vi "溶解氧电极校准.vi"() -> ()   [LabVIEW 2016, in "斯坦道多参数.lvlib"]
uses:
  <vilib>/Utility/miscctls.llb/LVPointTypeDef.ctl
  <vilib>/Analysis/NI_AALBase.lvlib
  <vilib>/ptbypt/NI_PtbyPt.lvlib
panel:
  out "标液2":string="饱和标准液"
  out "标液1":string="零点标准液"
  in  "刷新按钮":bool
  out "第二点信号值":dbl
  out "第一点信号值":dbl
  out "通讯状态":string
  out "第二点校准值":dbl
  out "第一点校准值":dbl
  out "最小值":sgl format="%#.2f"
  out "最大值":sgl format="%#.2f"
  in  "校准模式":enum16{"两点校准", "单点校准"}(ring)=enum."单点校准"
  in  "校准停止":bool
  in  "校准启动":bool
  out "波形图表":dbl(graph) caption="历史曲线"
  out "变异系数":dbl format="%#.6f"
  out "standard deviation":dbl caption="标准差" format="%#.2f"
  out "mean":dbl caption="均值" format="%#.2f"
  out "测量读值":dbl caption="测量值" format="%#.2f"
  out "偏移值补偿":dbl caption="溶解氧偏移修正值" format="%#.2f"
  out "饱和度值":dbl format="%#.2f"
  out "提示":string
  out "气压补偿值":dbl format="%#.2f"
  out "盐度补偿值":dbl format="%#.2f"
  out "电极斜率":dbl format="%#.6f"
  out "电极零点":dbl format="%#.6f"
  # "溶解氧电极设定"
  # "%"
  # "%"
  # "ppt"
  # "hPa"
  # "请选择校准模式:"
  # "mg/L"
  # "%"
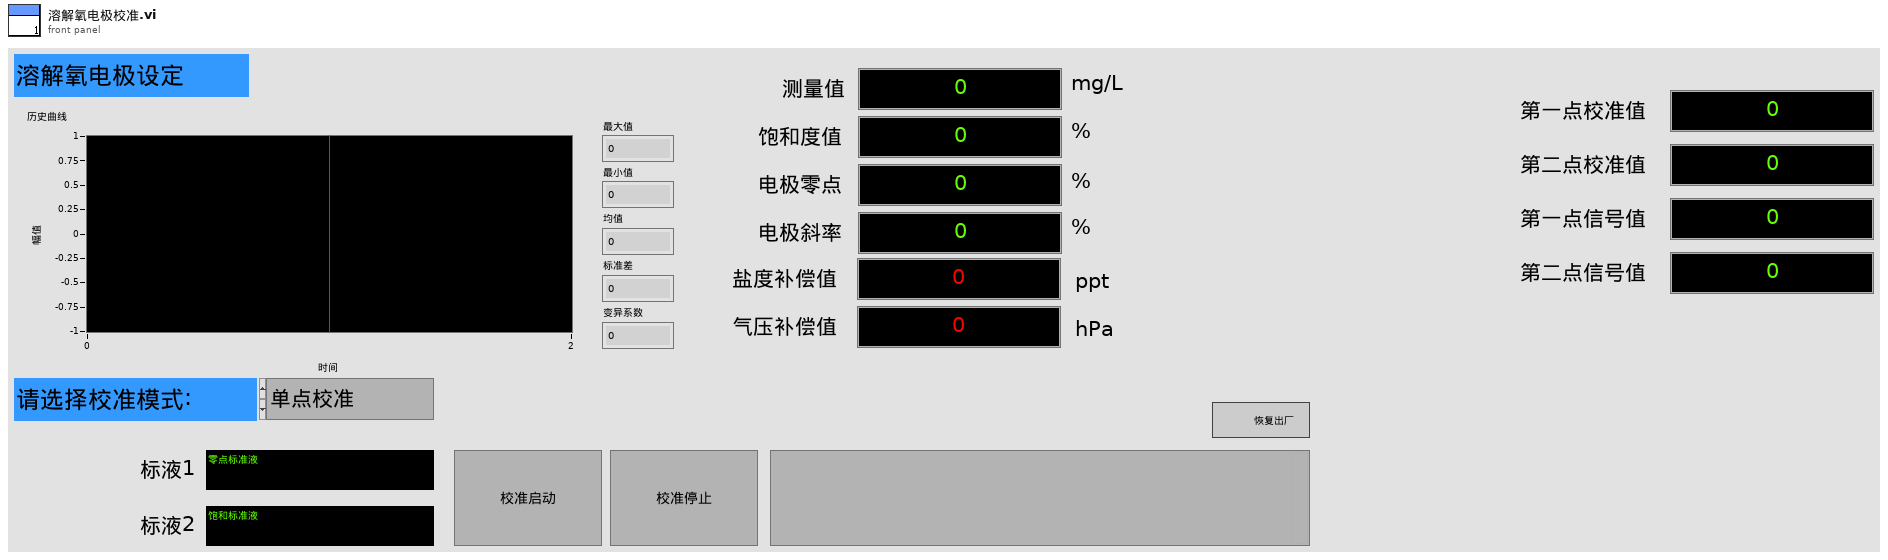
[diagram p1: front panel]
types:
  T1 = typedef "LVPointTypeDef.ctl" = cluster{"Horizontal":i16, "Vertical":i16}
  T2 = cluster{"电极状态标志":u16, "电极型号标志":u16, "溶解氧测量值":sgl, "温度测量值":sgl, "溶解氧饱和度值":sgl, "盐度补偿值":sgl, "大气压补偿值":sgl, "溶解氧偏移修正值":sgl, "温度偏移修正值":sgl, "手动温度补偿值":sgl, "溶解氧电极零点":sgl, "溶解氧电极斜率":sgl, "第1点标准值记录":sgl, "第1点信号值记录":sgl, "第1点温度值记录":sgl, "第2点标准值记录":sgl, "第2点信号值记录":sgl, "第2点温度值记录":sgl, "命令滤波设定":u16, "温度模式":enum16{"ATC", "MTC"}, "生产批次":u16, "电极序号":u16, "串口地址":u16, "串口波特率":enum16{"9600", "19200", "115200"}, "串口校验位":enum16{"NONE", "ODD", "EVEN"}, "串口停止位":enum16{"1bit", "2bit"}, "第一点标准值":sgl, "第二点标准值":sgl}
  T3 = enum8{"Enabled", "Disabled", "Disabled and Grayed Out"}
  T4 = cluster{"ph":bool, "DO":bool, "Cond":bool, "Turb":bool, "叶绿素a":bool, "藻密度":bool, "ORP":bool}
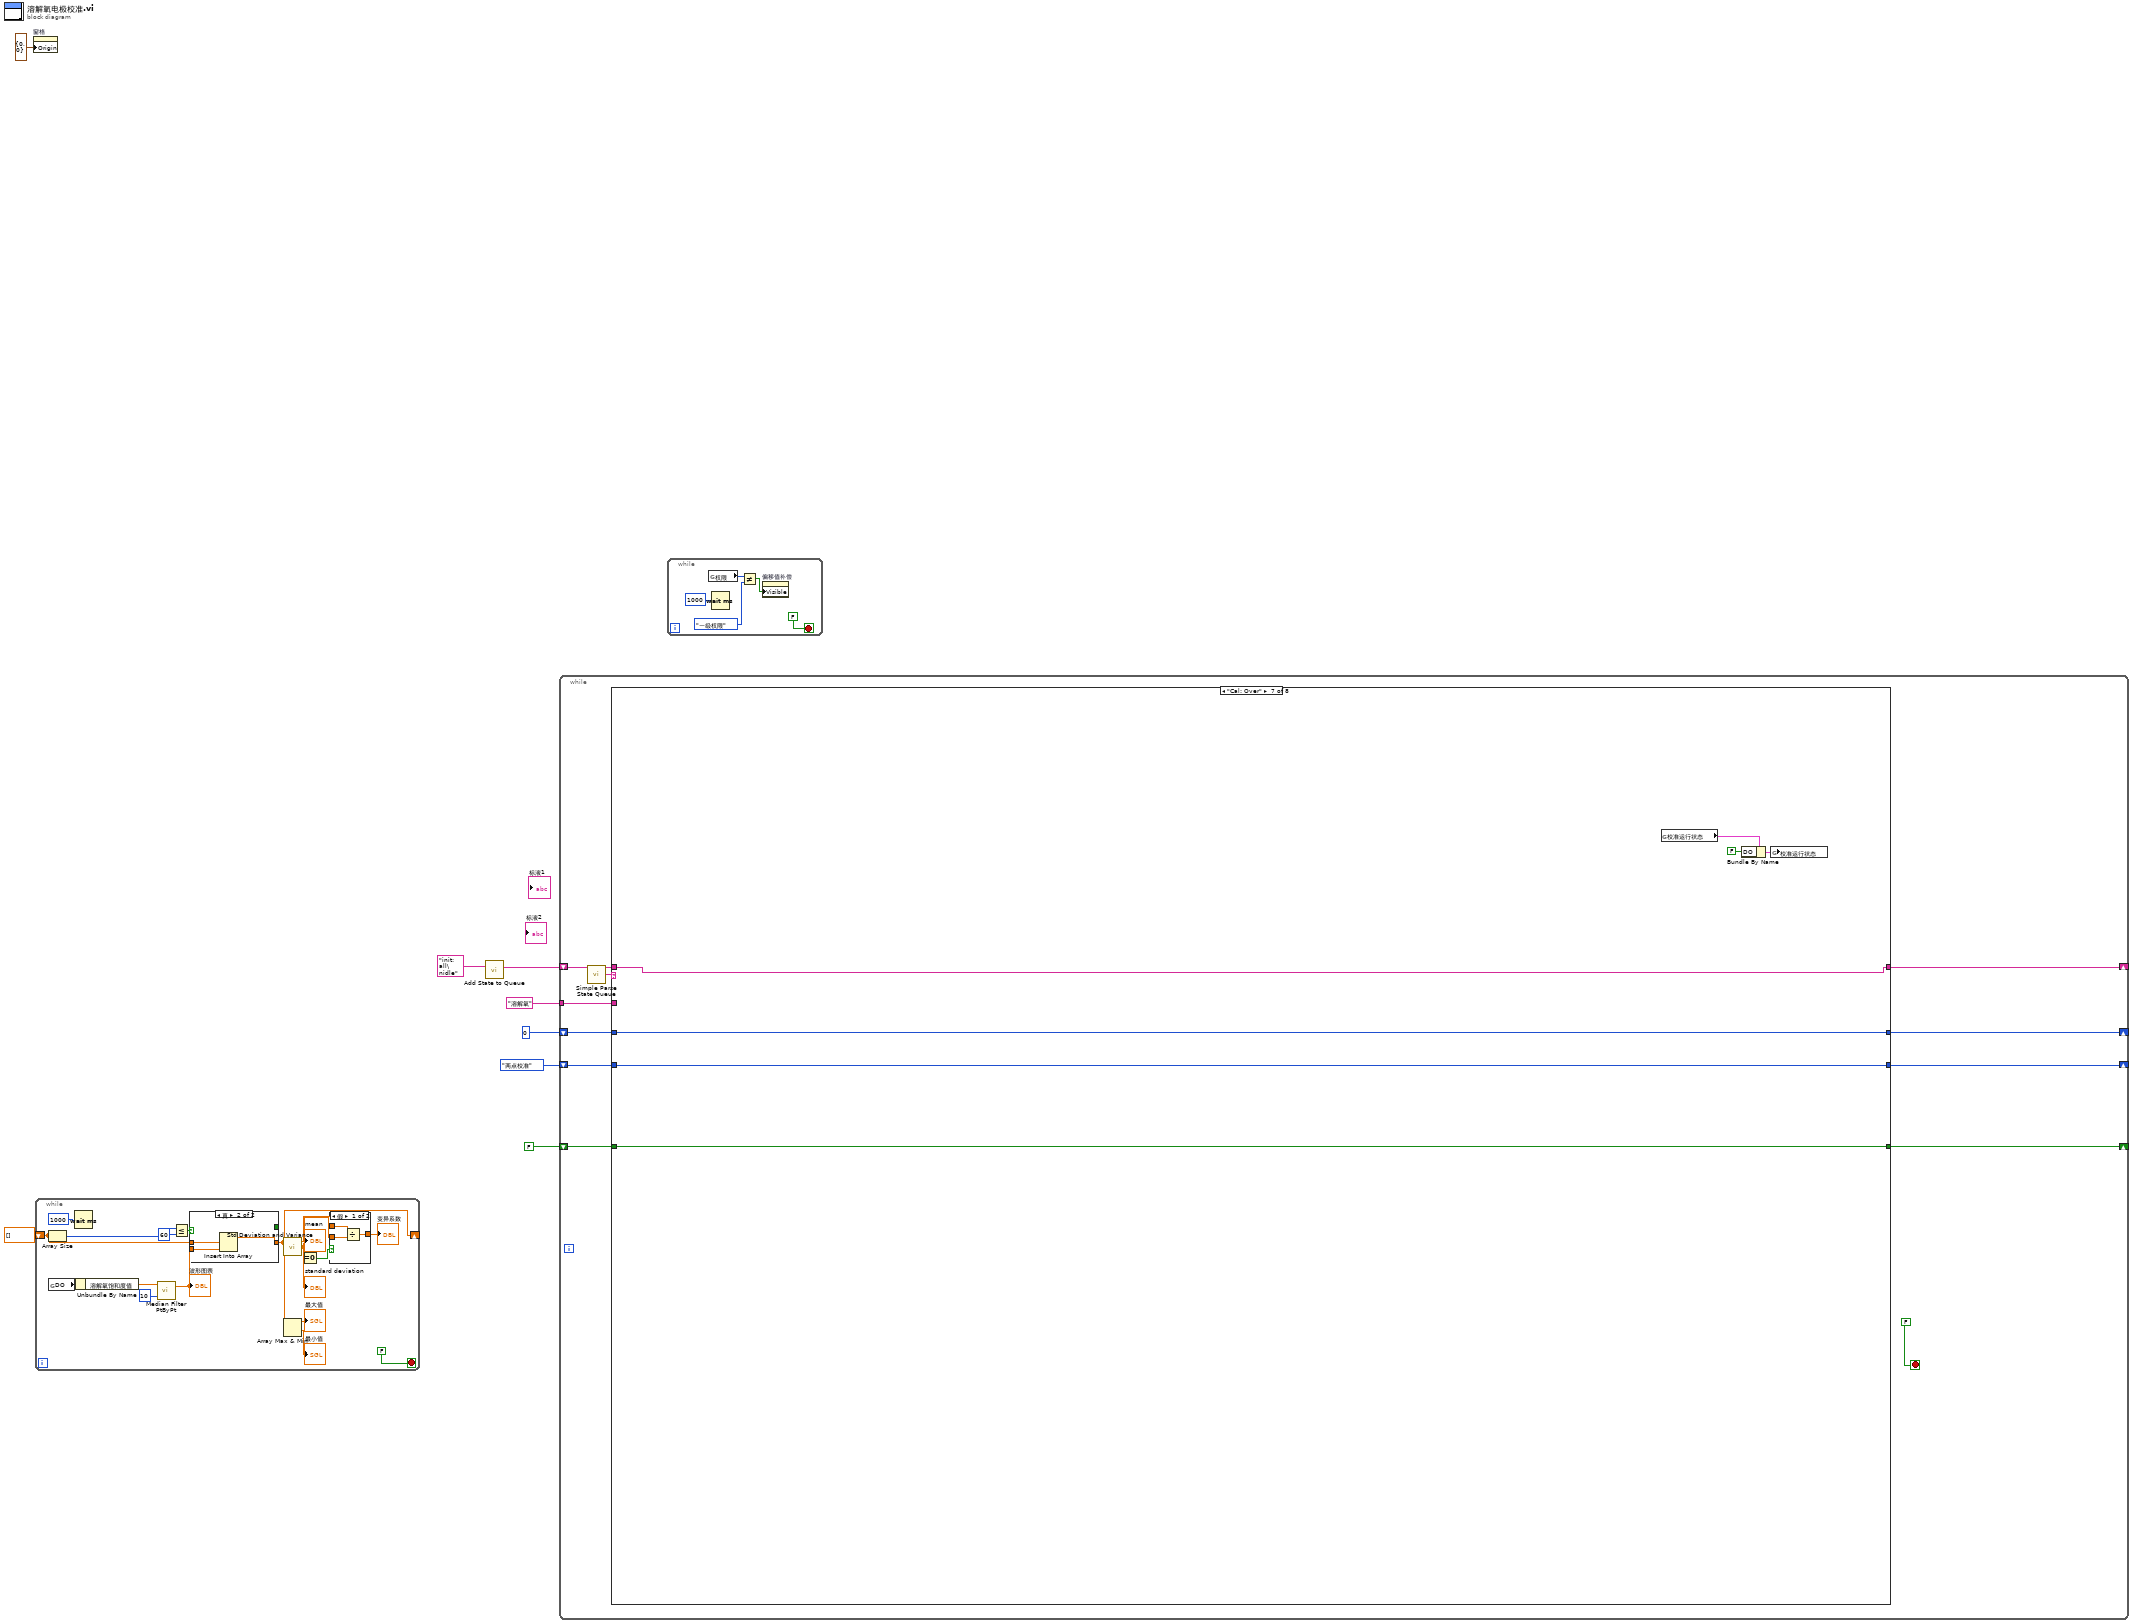
[diagram p0: block diagram]
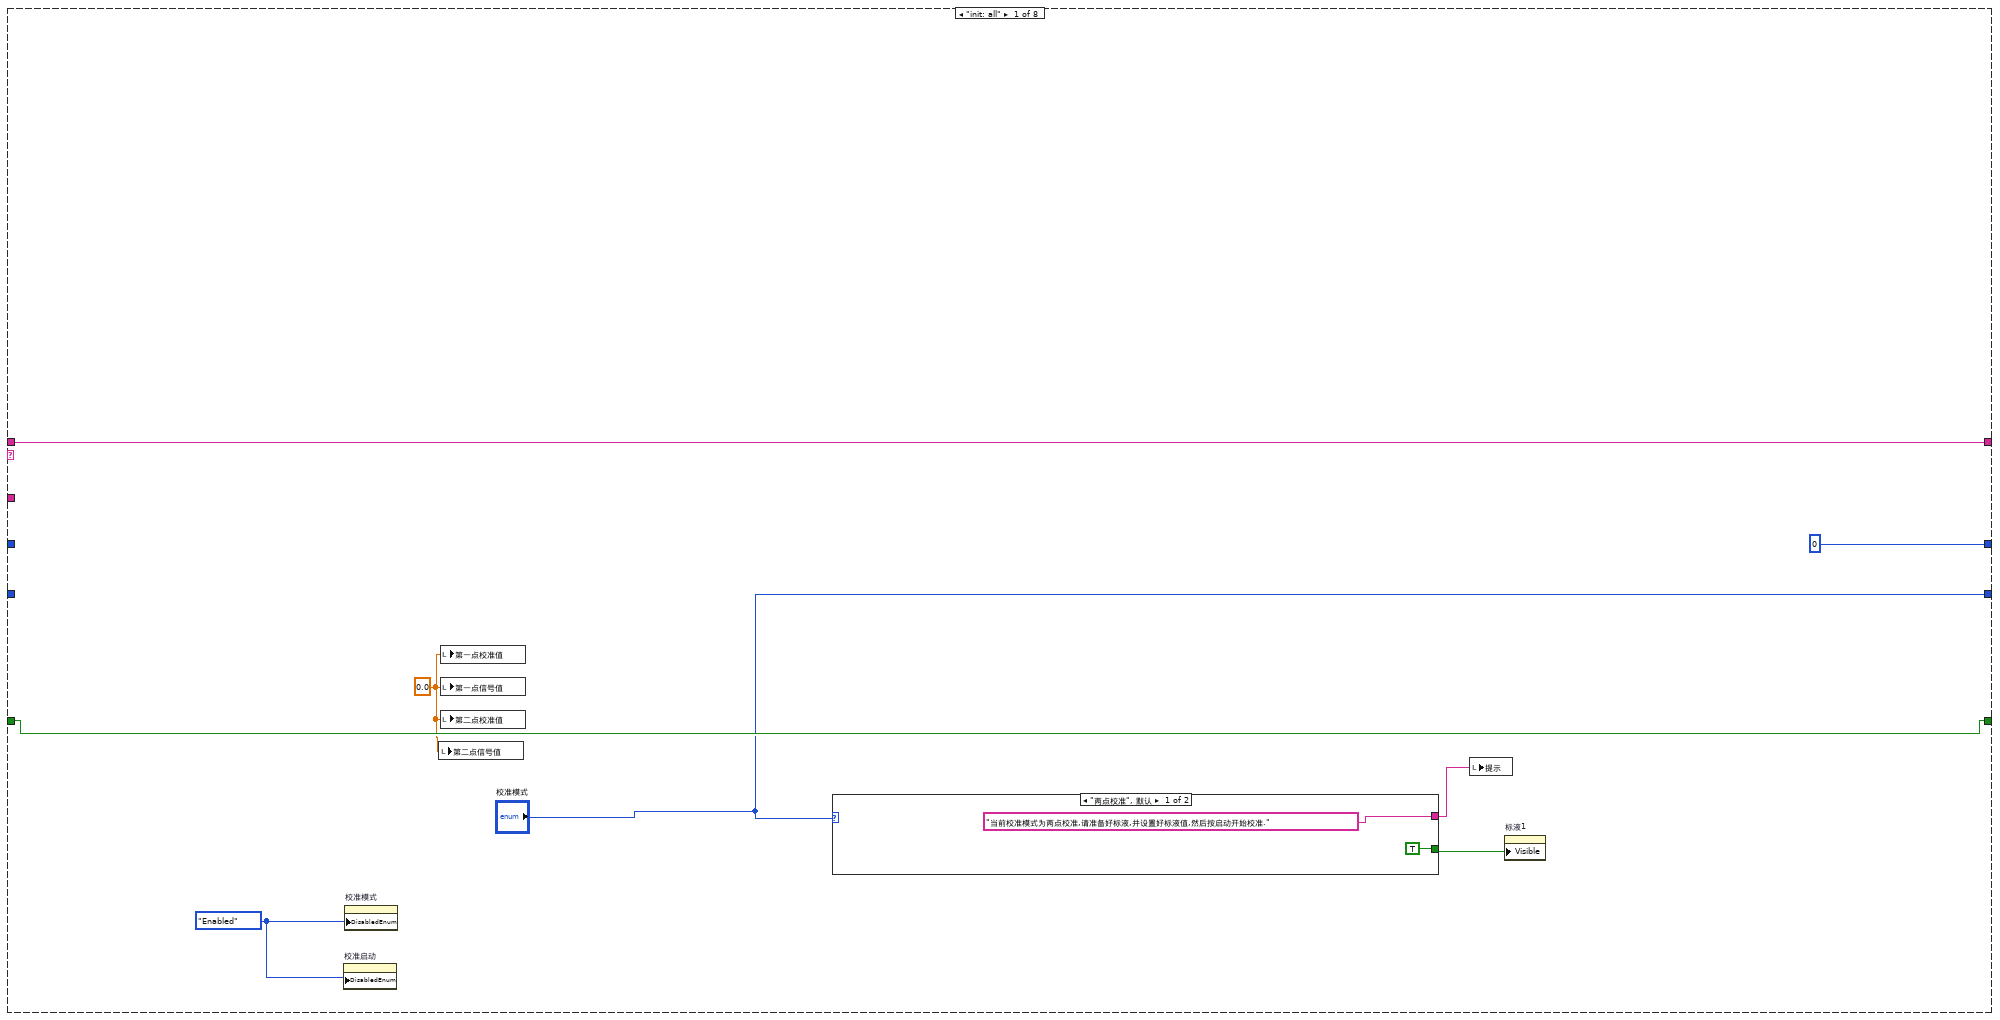
[diagram p2: hidden frame]
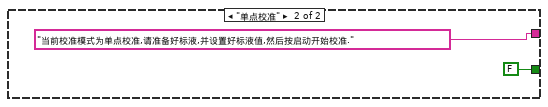
[diagram p3: hidden frame]
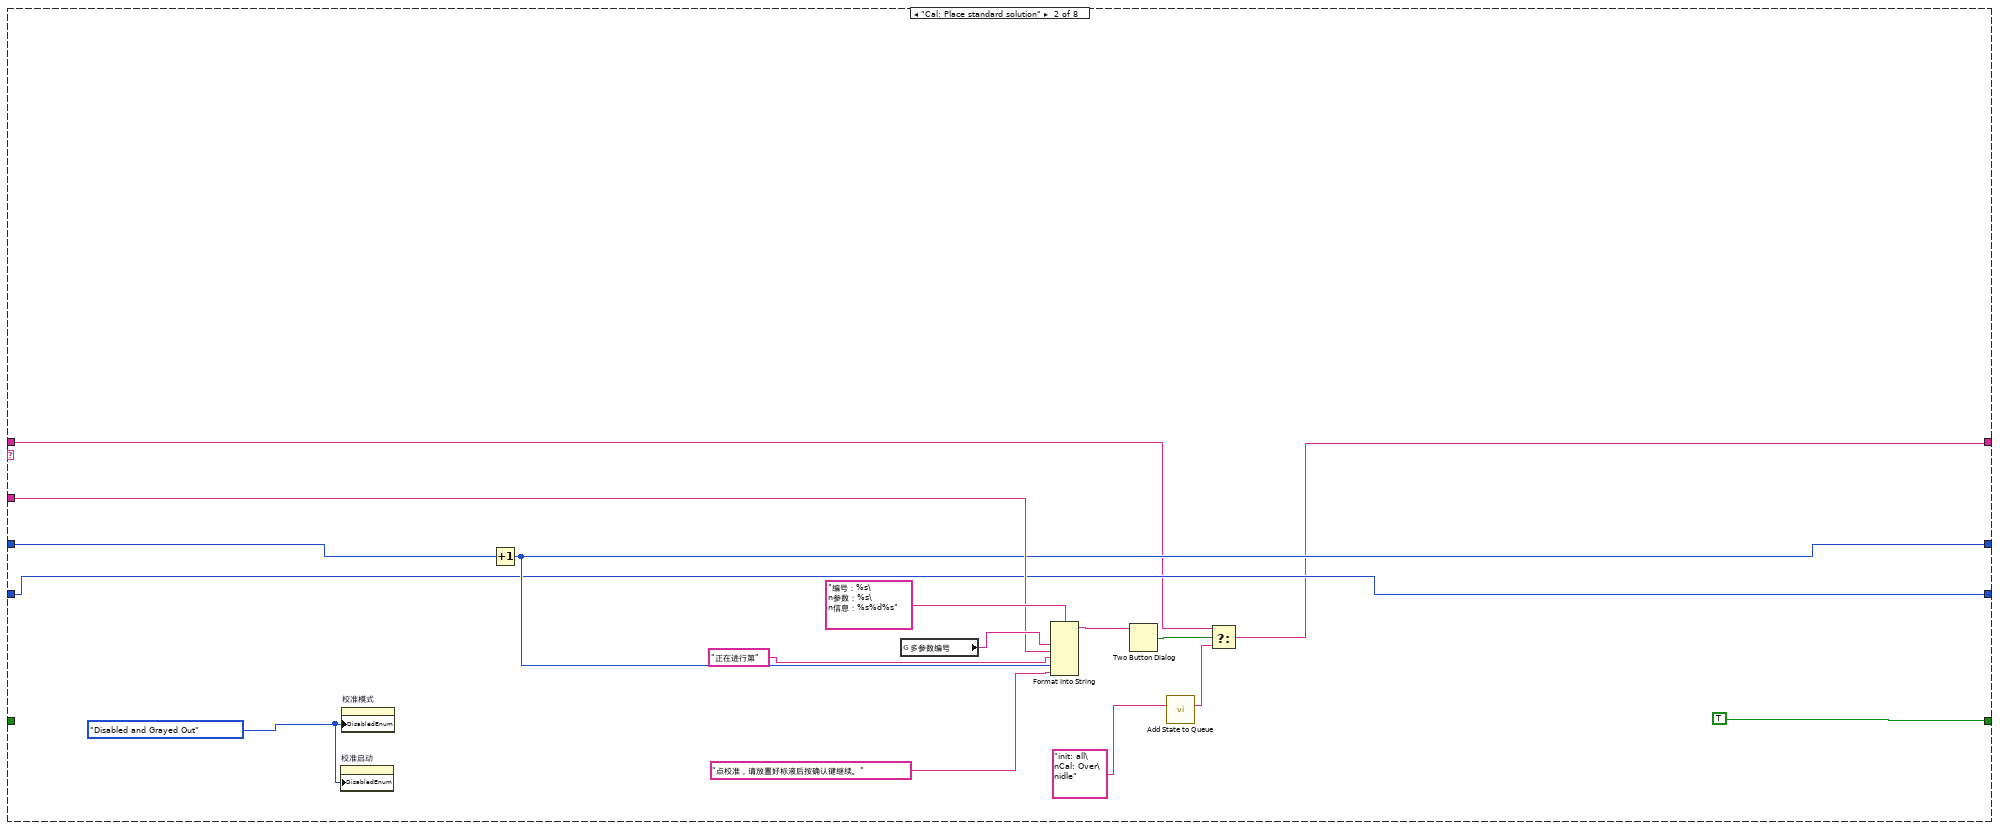
[diagram p4: hidden frame]
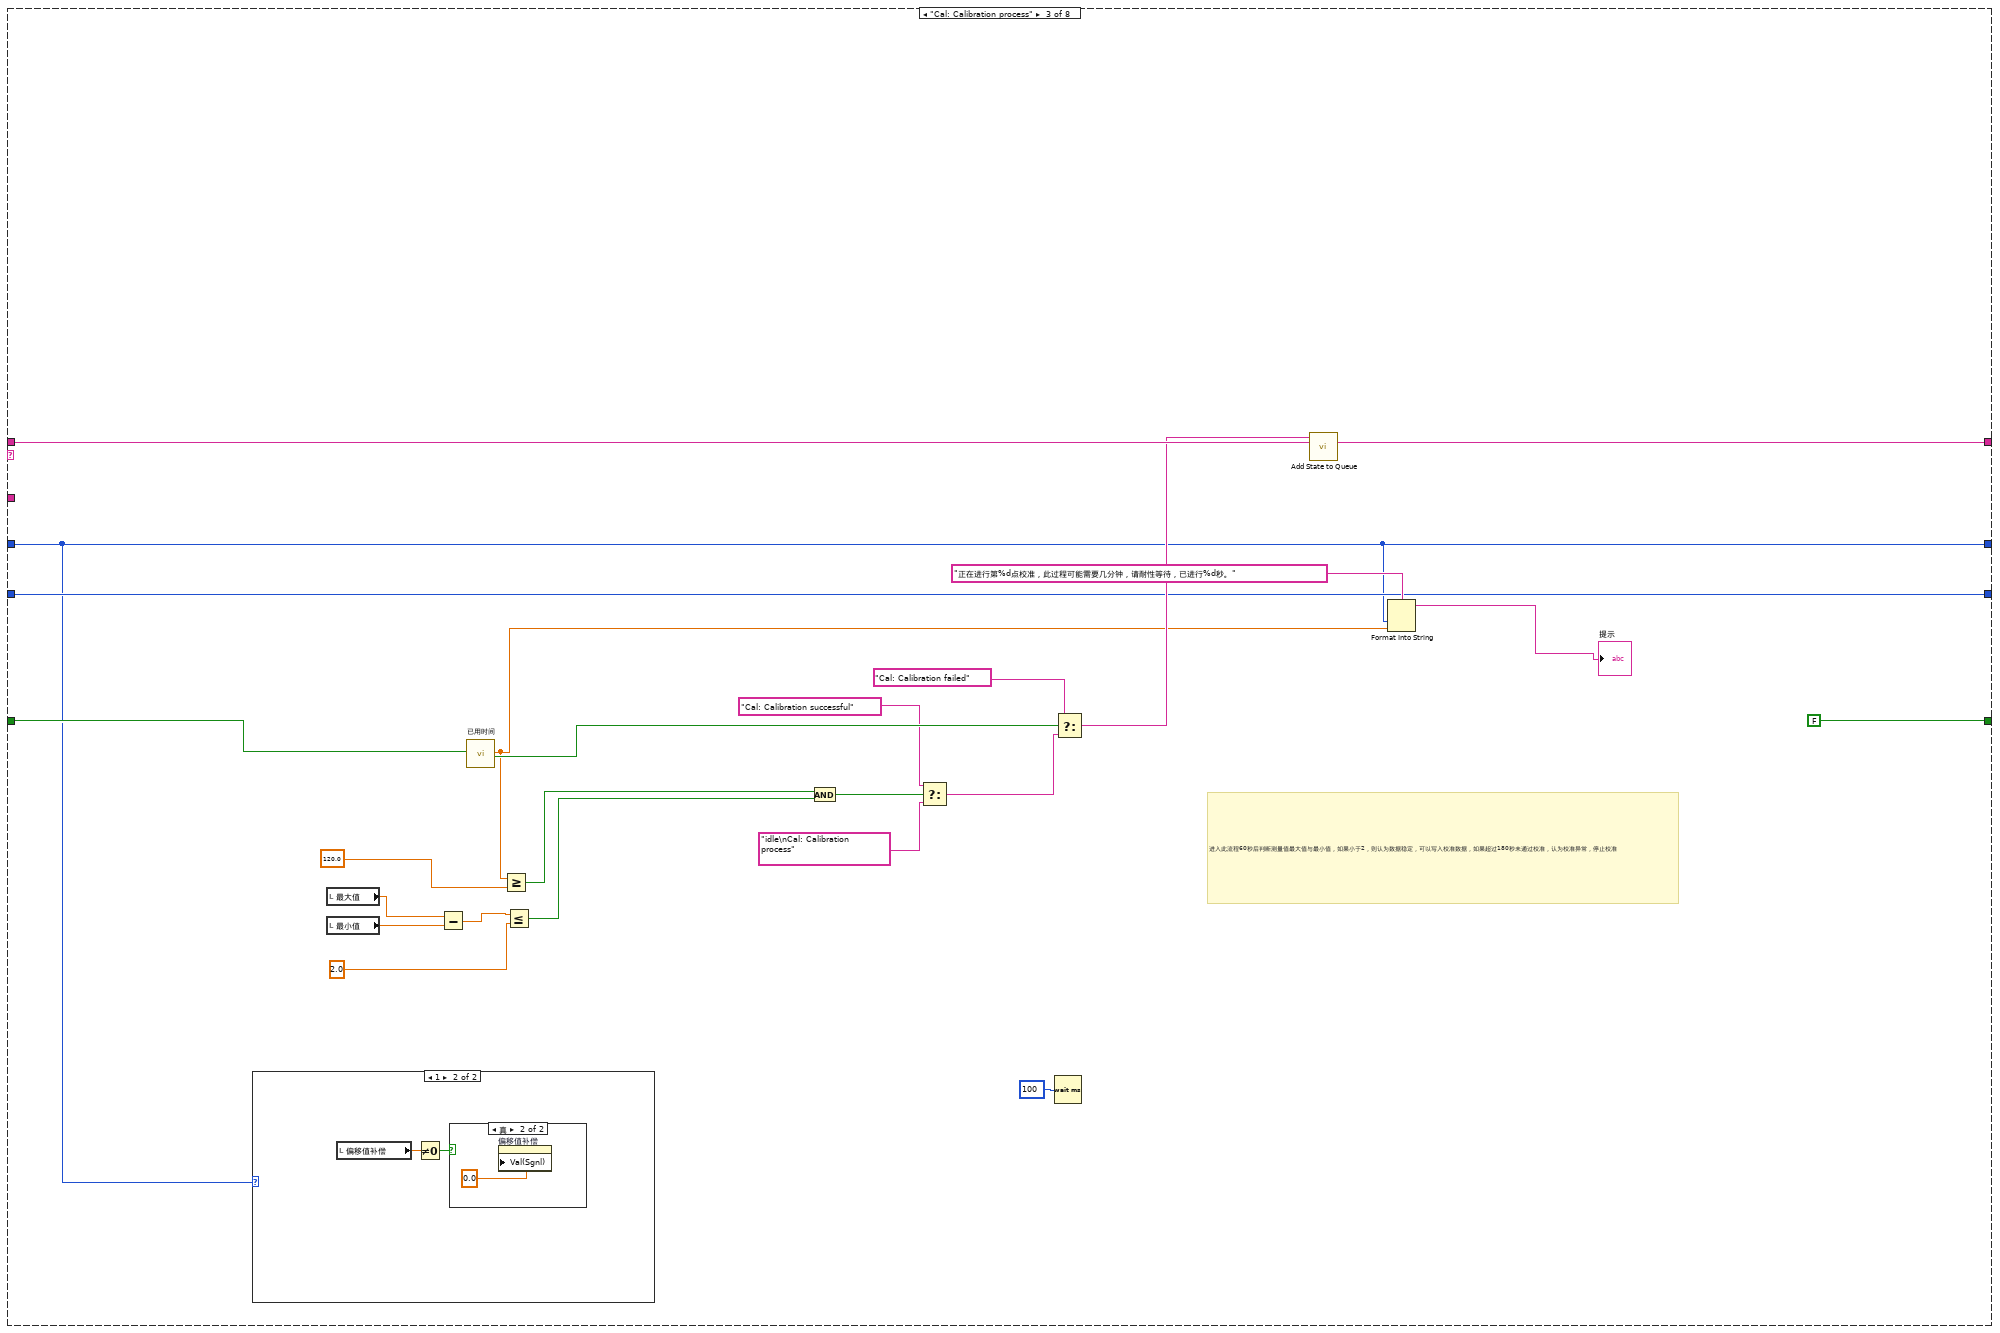
[diagram p5: hidden frame]
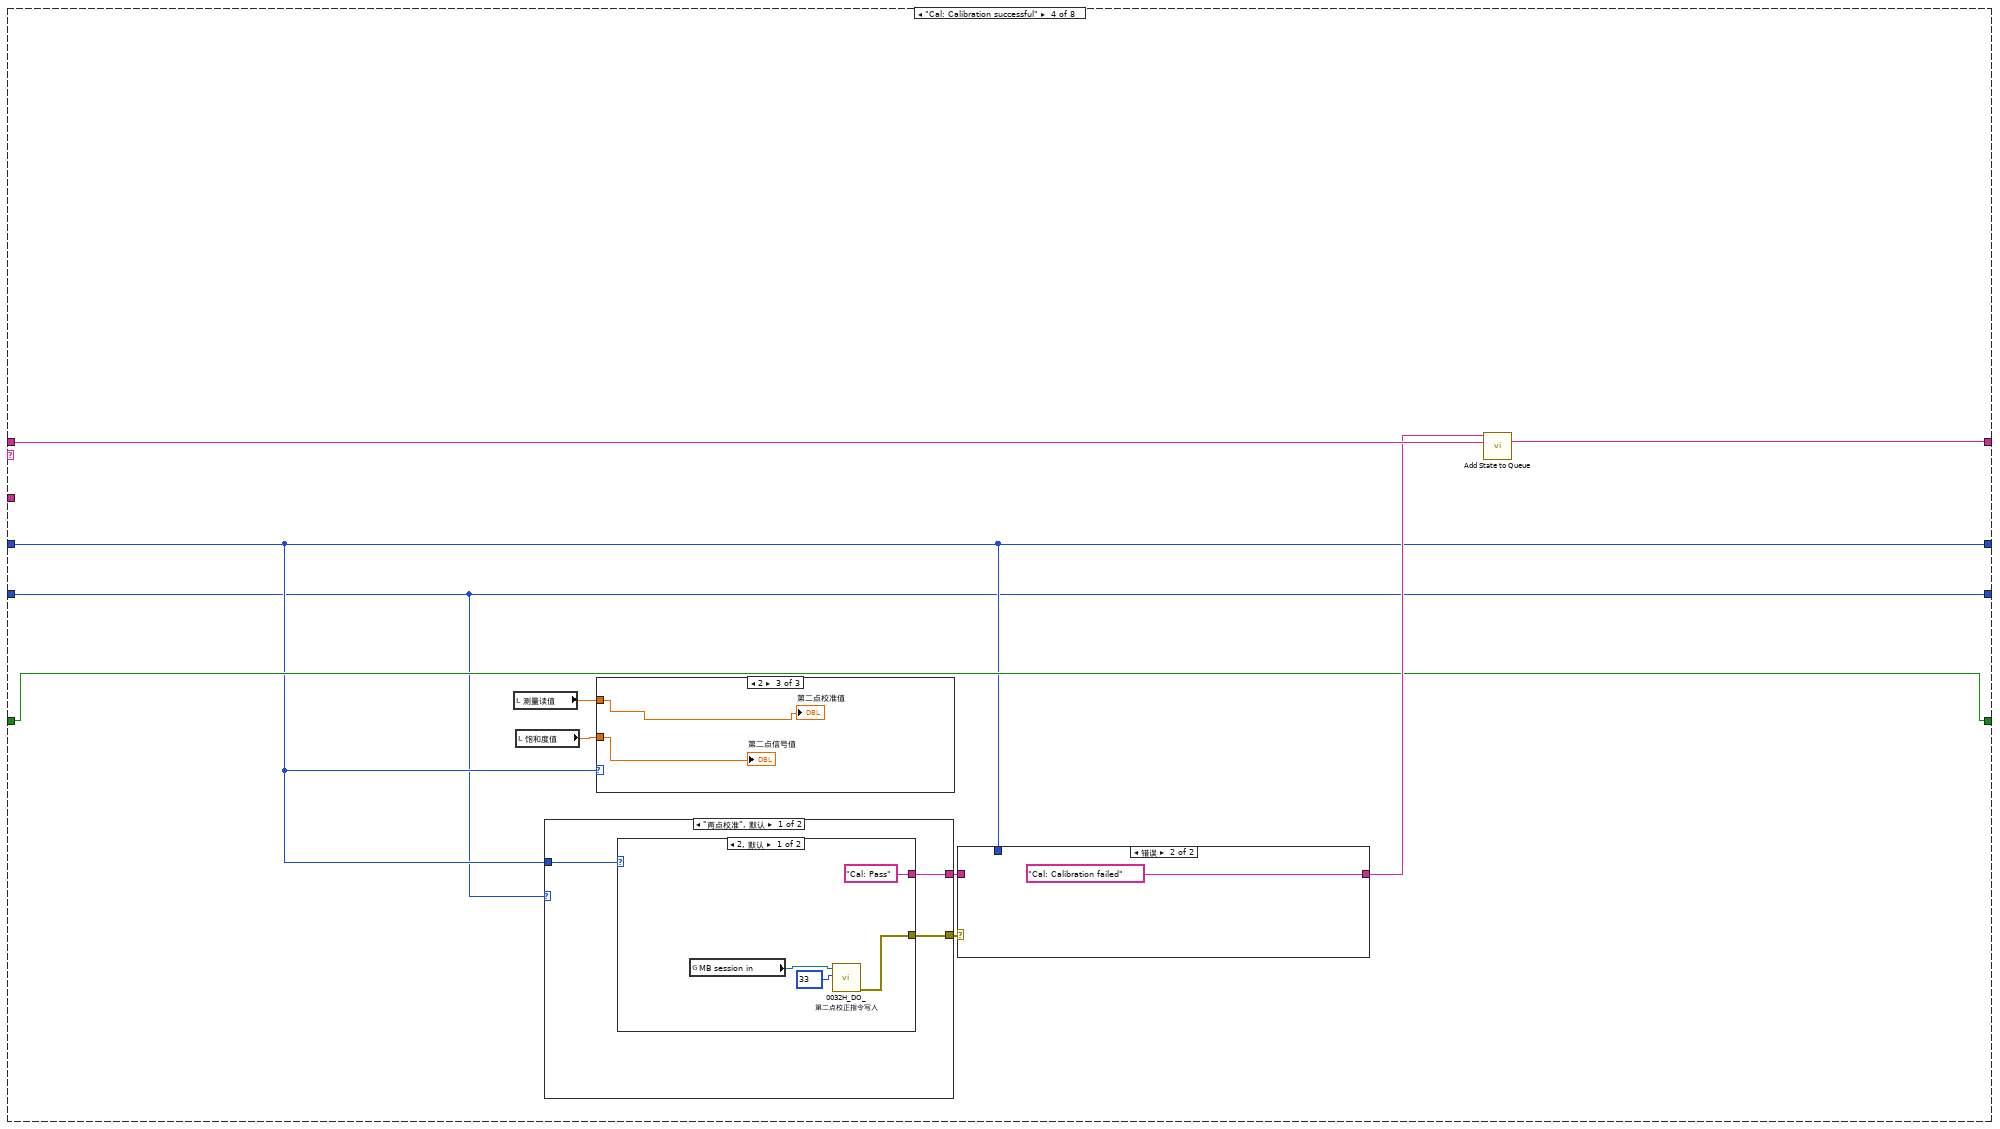
[diagram p8: hidden frame]
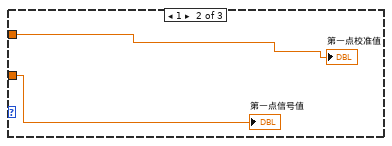
[diagram p10: hidden frame]
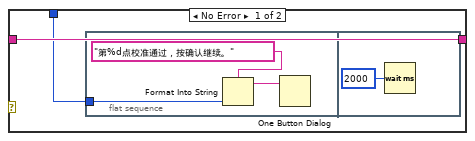
[diagram p11: hidden frame]
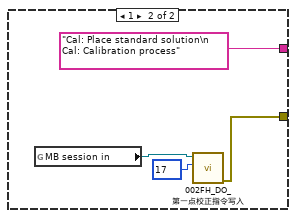
[diagram p12: hidden frame]
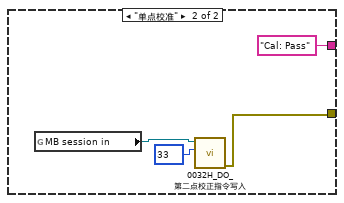
[diagram p13: hidden frame]
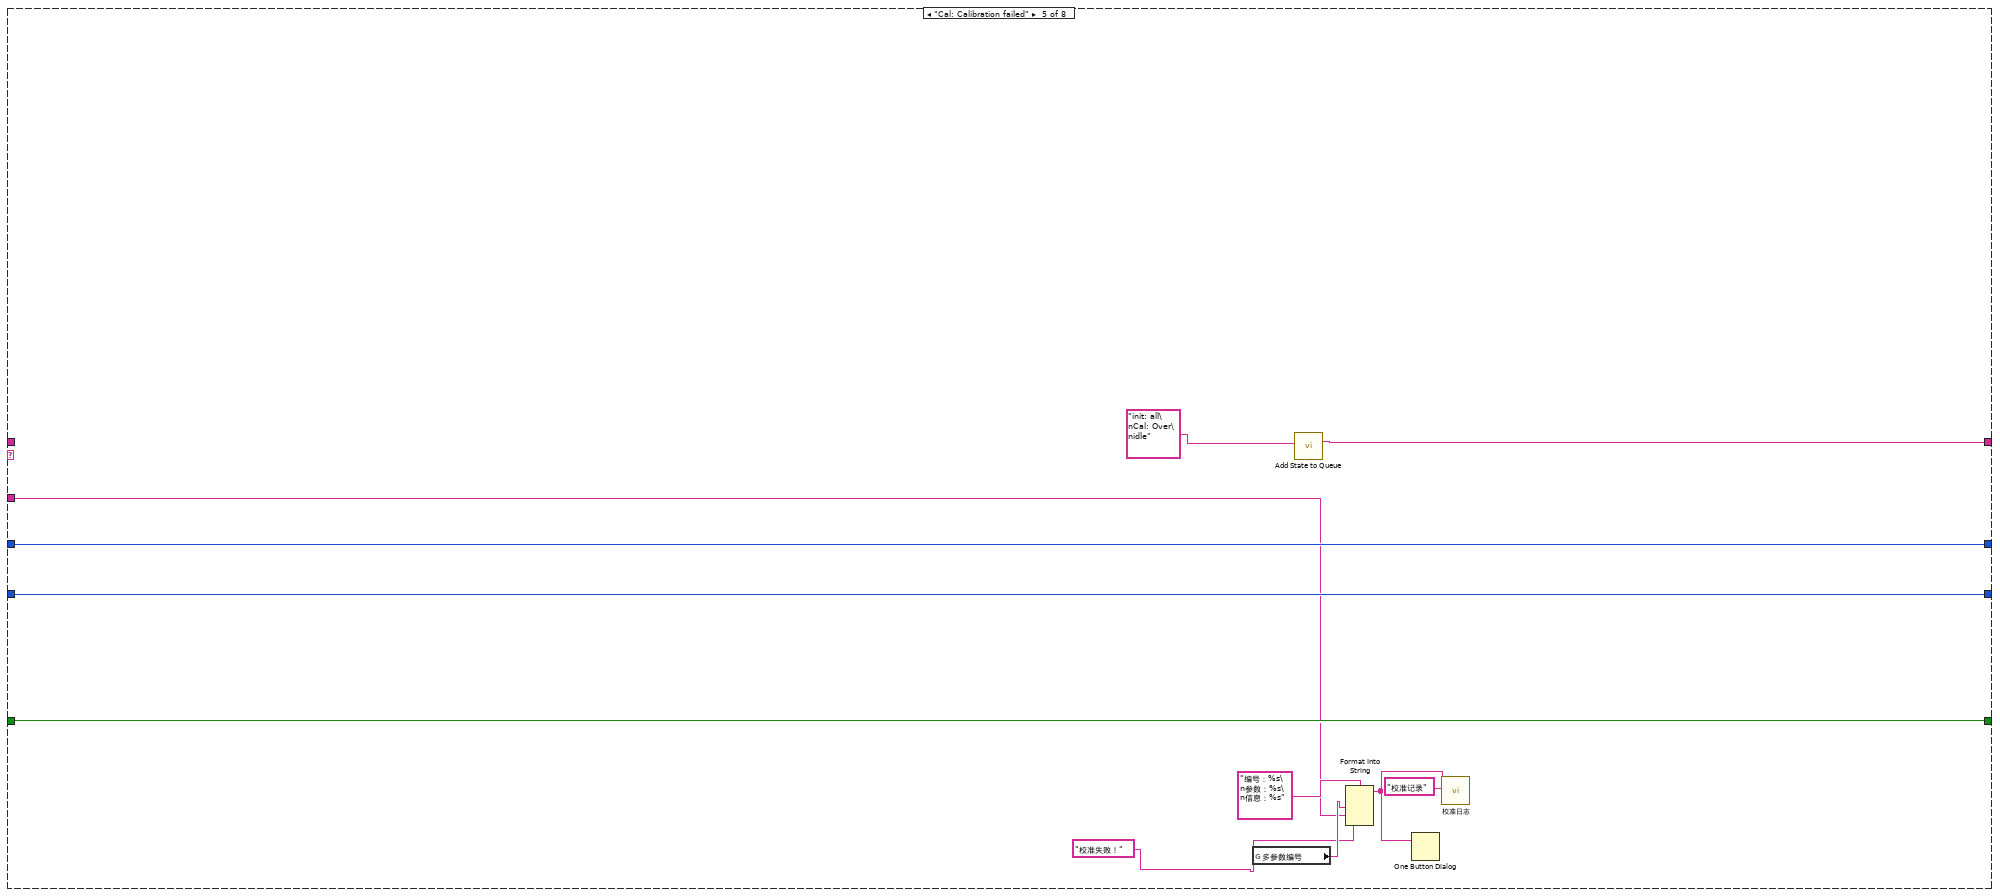
[diagram p14: hidden frame]
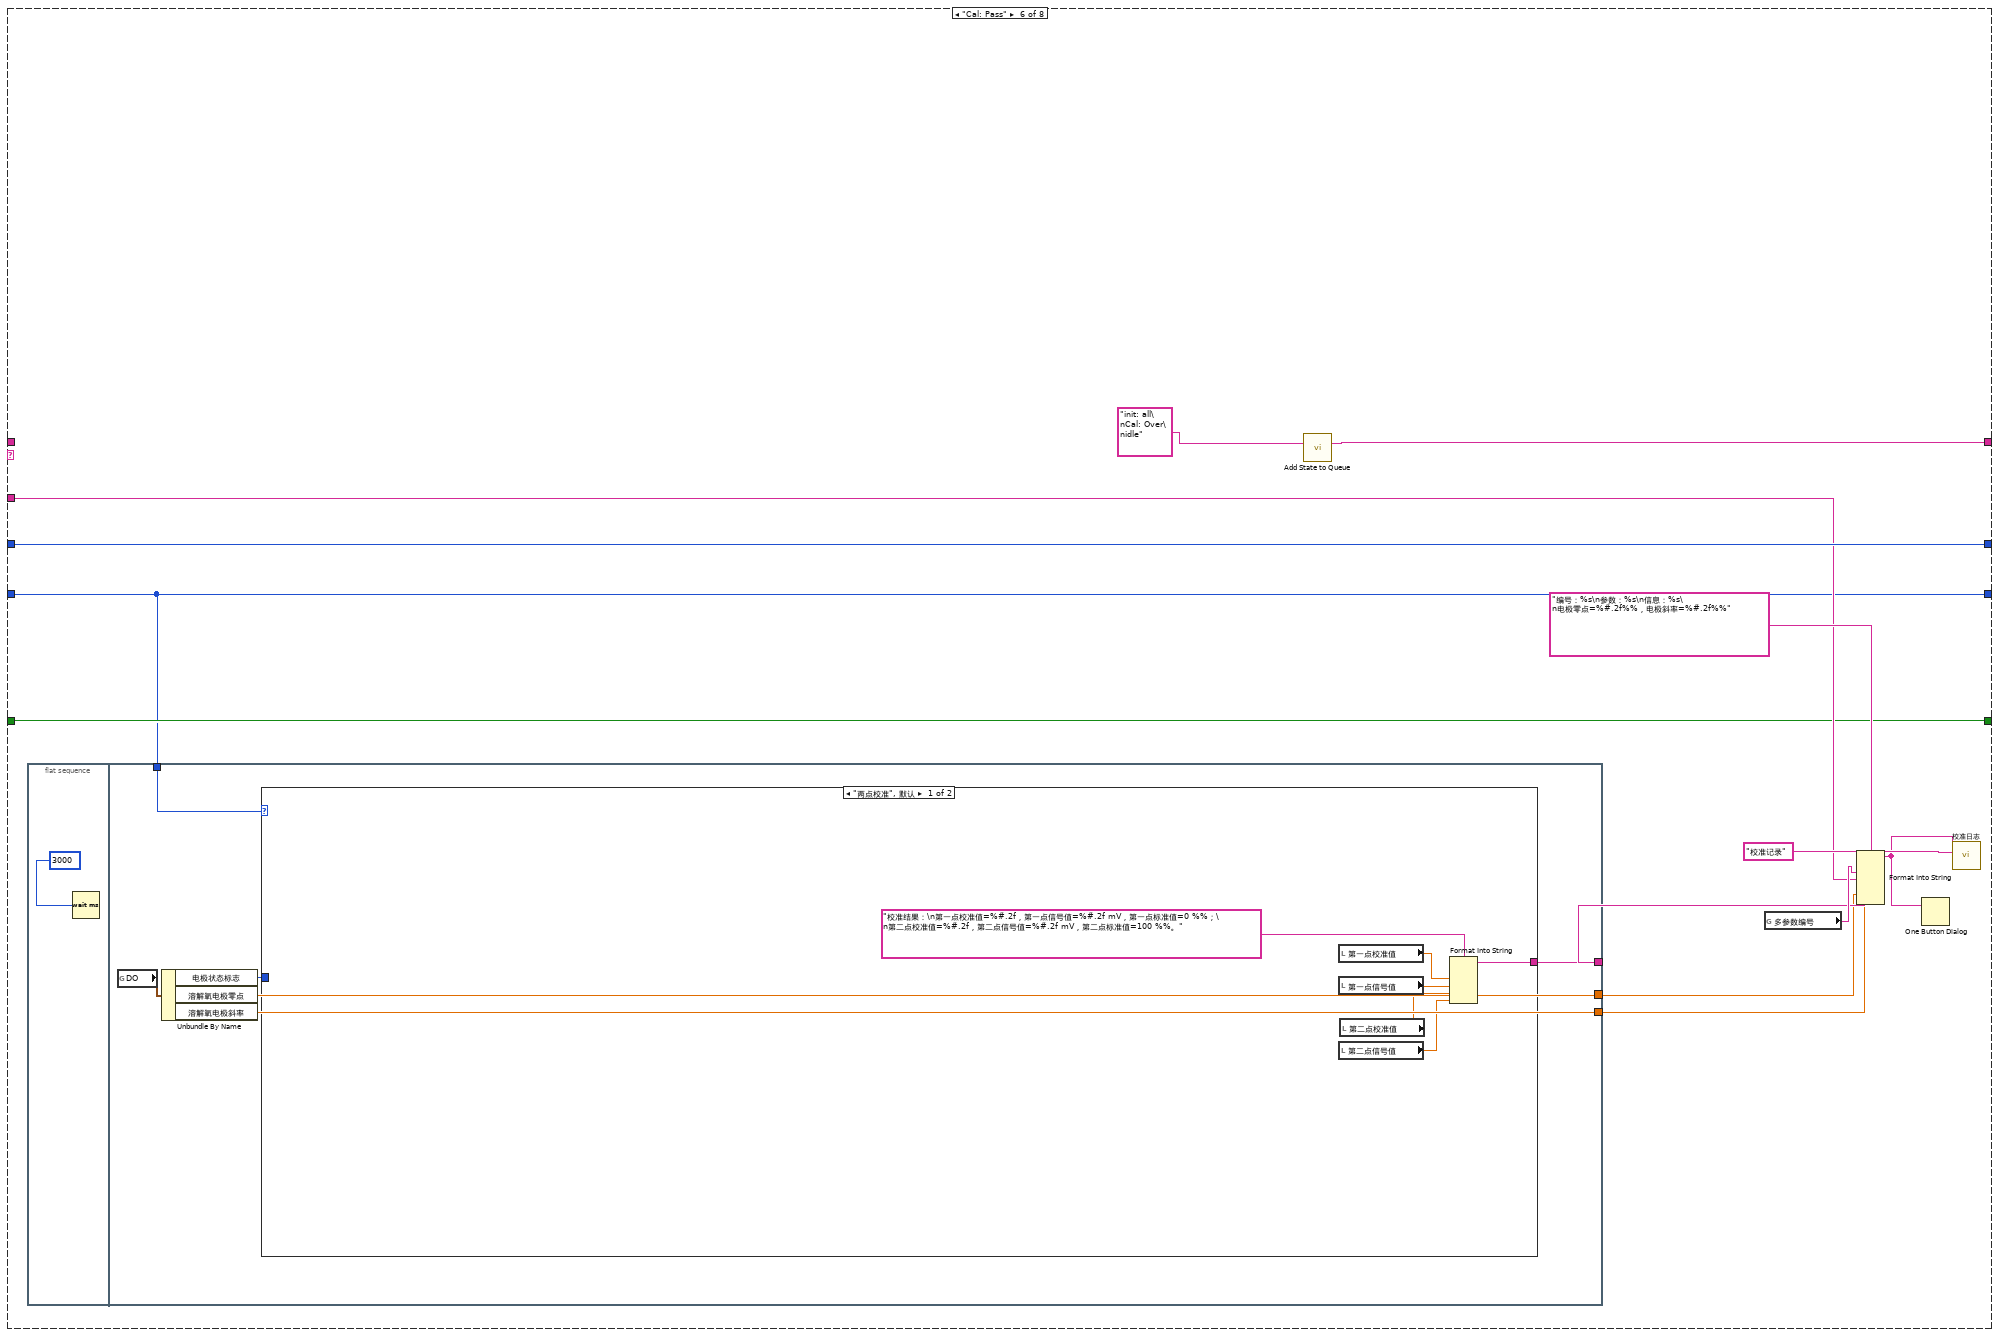
[diagram p15: hidden frame]
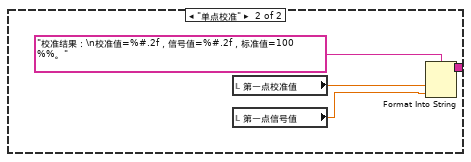
[diagram p16: hidden frame]
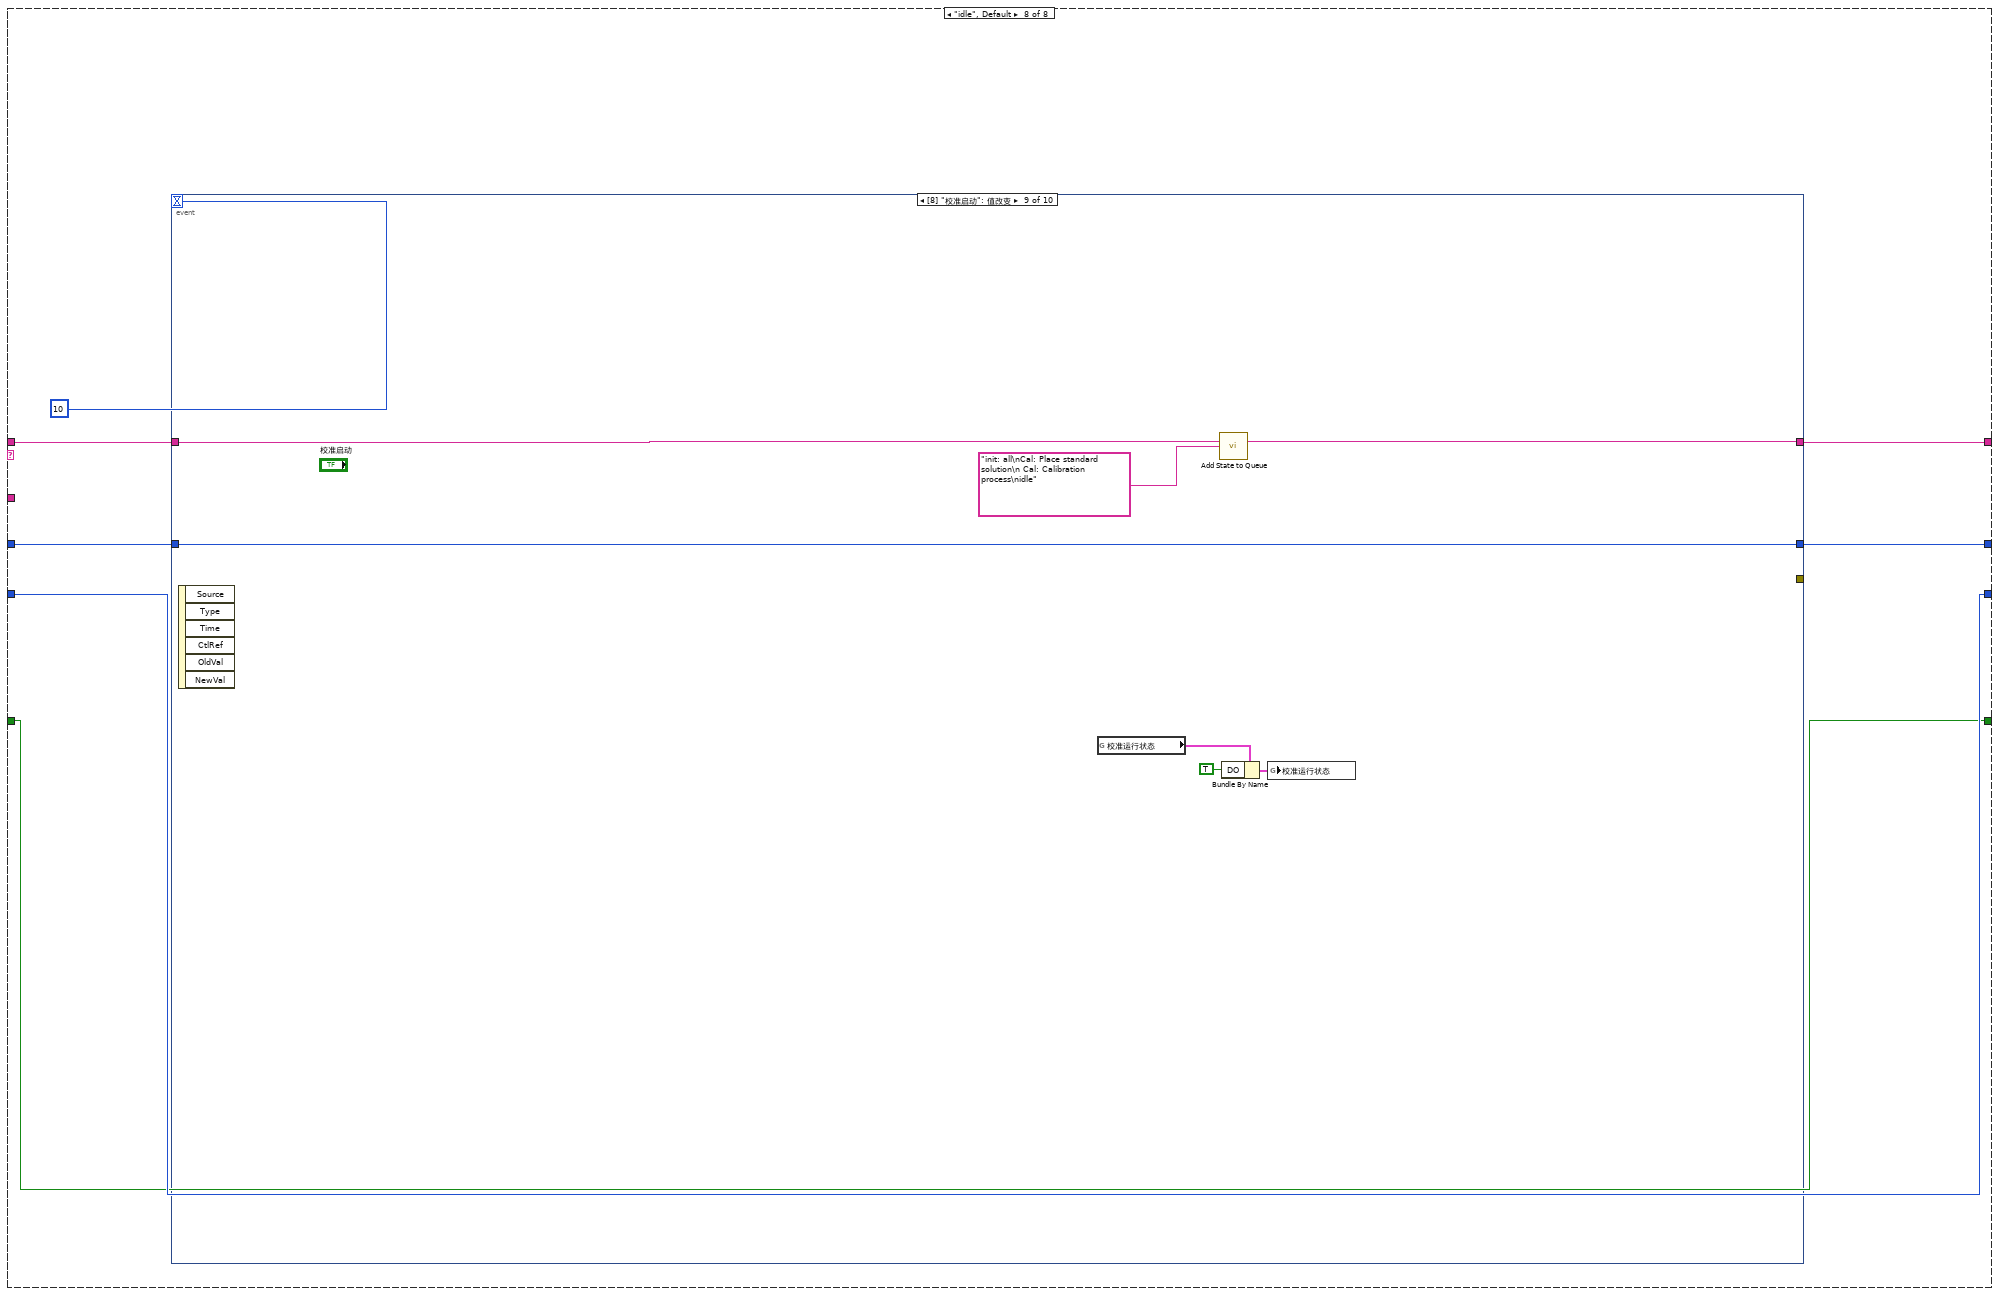
[diagram p17: hidden frame]
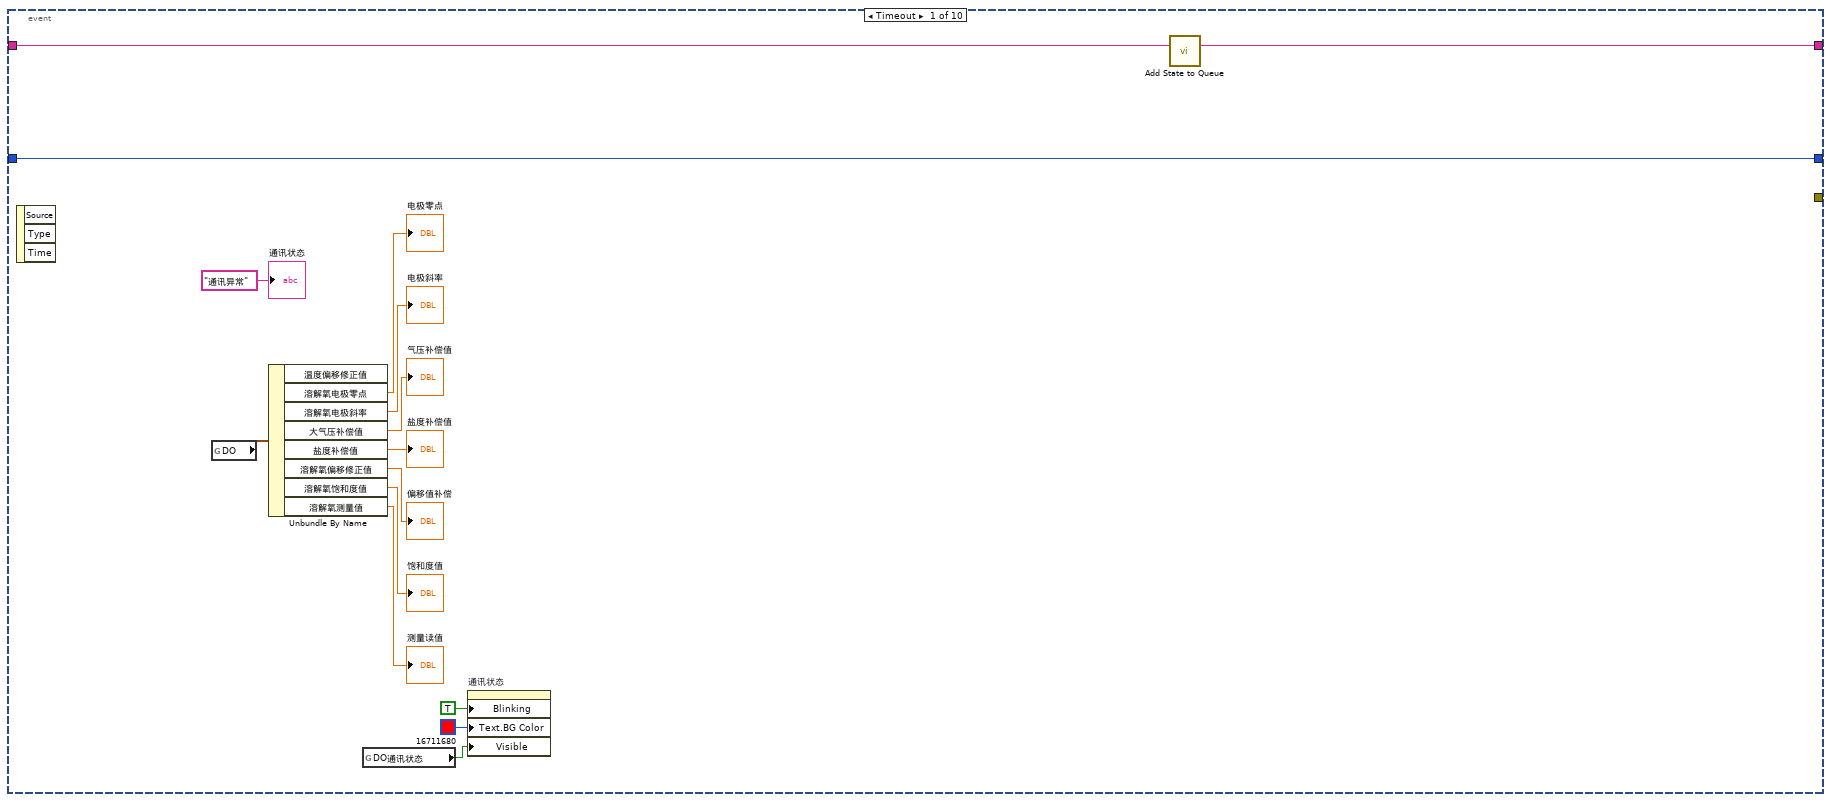
[diagram p18: hidden frame]
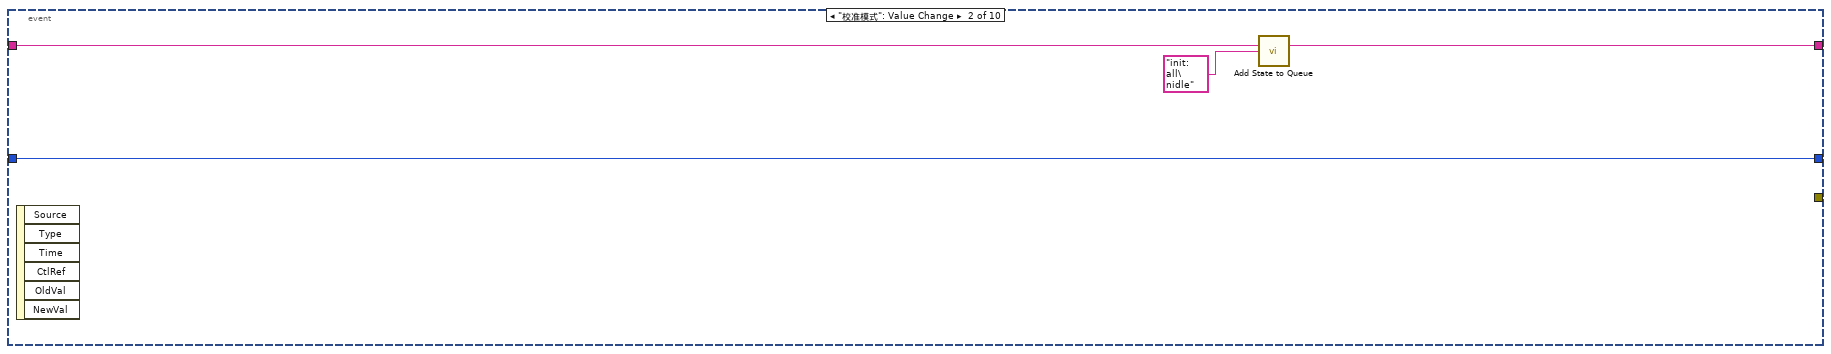
[diagram p19: hidden frame]
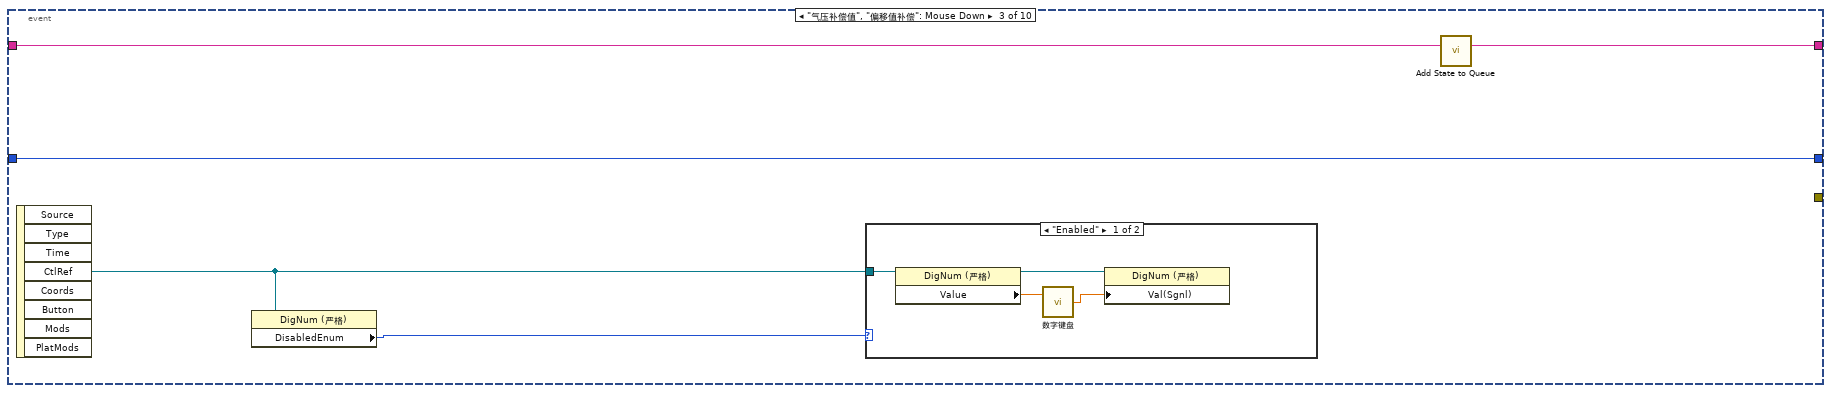
[diagram p20: hidden frame]
diagram:
  n1 = property on="窗格" class="Pane"("Origin"=T1 {"Horizontal"=0, "Vertical"=0} ("原点")) -> ()  [unwired: 2 in, 2 out]
  n2 = while {
    shift-right: [w14] -> _
    shift-left: sgl[] [] -> [w21]
    stop <- FALSE stop-if-true
    n3 = Array Size(array=w21) -> (size(s)=w23:i32)
    n4 = global read "国弘过程全局变量.vi" "DO"() -> (w17:T2)
    n5 = Wait (ms)(milliseconds to wait=u32 1000 ("等待时间（毫秒）")) -> ()  [unwired: 1 out]
    n6 = Unbundle By Name(w17) -> ("溶解氧饱和度值"=w10:sgl)
    n7 = call <vilib>:"Median Filter PtByPt.vi"("rank"=10, "x"=w10) -> ("Filtered x"=w9:dbl)  [unwired: 2 in, 1 out]
    "波形图表" <- w9
    n8 = Less Or Equal?(x=w23, y=60) -> (x <= y?=w22:bool)
    n9 = case shown="真" w22 {
      tunnel: w21 -> [w34 w37]
      tunnel: w9 -> [w32 w36]
      tunnel: [w30 w35] -> w14
      tunnel: [TRUE _] -> _
      frame False {
        n10 = Replace Array Subset(array=w34, new element=w32) -> (w33:sgl[])  [unwired: 1 in]
        n11 = Rotate 1D Array(1:w33, 2:-1 ("n")) -> (0:w30:sgl[])
      }
      frame True {
        n12 = Insert Into Array(array=w37, new element=w36) -> (w35:sgl[])  [unwired: 1 in]
      }
    }
    n13 = call <vilib>:"Std Deviation and Variance.vi"("X"=w14) -> ("mean"=w16:dbl, "standard deviation"=w15:dbl)  [unwired: 1 in, 1 out]
    "mean" <- w16
    "standard deviation" <- w15
    n14 = Array Max & Min(array=w14) -> (max value=→"最大值":sgl, min value=→"最小值":sgl)  [unwired: 2 out]
    n15 = Equal To 0?(x=w16) -> (x = 0?=w20:bool)
    n16 = case shown="假" w20 {
      tunnel: w15 -> [w28 _]
      tunnel: [w27 _] -> w19
      tunnel: w16 -> [w26 _]
      frame False {
        n17 = Divide(x=w28, y=w26) -> (x/y=w27:dbl)
      }
      frame True {
      }
    }
    "变异系数" <- w19
  }
  n18 = call "Add State to Queue.vi"("State(s) In (\"\")"="init: all\nidle" ("State(s) In (\"\")")) -> ("States Out"=w5:string)  [unwired: 14 in]
  n19 = while {
    shift-right: [w45] -> _
    shift-left: w5 -> [w49]
    shift-right: [w42] -> _
    shift-left: 0 -> [w44]
    tunnel: "溶解氧" ("State(s) In (\"\")") -> [w43]
    shift-right: [w40] -> _
    shift-left: enum16{"两点校准", "单点校准"}."两点校准" ("校准模式") -> [w41]
    shift-right: [w38] -> _
    shift-left: FALSE -> [w39]
    stop <- FALSE stop-if-true
    n20 = call "Simple Parse State Queue.vi"("State Queue"=w49) -> ("Remain States"=w46:string, "Next State"=w47:string)  [unwired: 13 in]
    n21 = case shown="\"Cal: Over\"" w47 {
      tunnel: w46 -> [w57 w65 w96 w112 _ _ w188 w195]
      tunnel: [w57 w64 w95 w111 w148 w155 w188 w194] -> w45
      tunnel: w44 -> [_ w73 w80 w106 w151 w164 w187 w192]
      tunnel: w43 -> [_ w74 _ _ w142 w160 _ _]
      tunnel: [0 w71 w80 w106 w151 w164 w187 w193] -> w42
      tunnel: w41 -> [_ w70 w81 w105 w150 w156 w186 w191]
      tunnel: ["校准模式" w70 w81 w105 w150 w156 w186 w191] -> w40
      tunnel: w39 -> [w54 _ w83 w107 w149 w159 w185 w189]
      tunnel: [w54 TRUE FALSE w107 w149 w159 w185 w189] -> w38
      frame "init: all" {
        w52 = T3."Enabled" ("禁用")
        w53 = 0.0 ("第一点校准值")
        n22 = property on="校准启动" class="Bool"("DisabledEnum"=w52) -> ()  [unwired: 2 in, 2 out]
        n23 = property on="校准模式" class="Enum (严格)"("DisabledEnum"=w52) -> ()  [unwired: 2 in, 2 out]
        n24 = local write "第二点信号值"(w53) -> ()
        n25 = local write "第一点校准值"(w53) -> ()
        n26 = local write "第一点信号值"(w53) -> ()
        n27 = local write "第二点校准值"(w53) -> ()
        n28 = case shown="\"两点校准\", 默认" "校准模式" {
          tunnel: ["当前校准模式为两点校准,请准备好标液,并设置好标液值,然后按启动开始校准." ("提示") "当前校准模式为单点校准,请准备好标液,并设置好标液值,然后按启动开始校准." ("提示")] -> w56
          tunnel: [TRUE ("可见") FALSE ("可见")] -> w50
          frame "两点校准", Default {
          }
          frame "单点校准" {
          }
        }
        n29 = local write "提示"(w56) -> ()
        n30 = property on="标液1" class="Str"("Visible"=w50) -> ()  [unwired: 2 in, 2 out]
      }
      frame "Cal: Place standard solution" {
        w63 = T3."Disabled and Grayed Out" ("禁用")
        n31 = property on="校准启动" class="Bool"("DisabledEnum"=w63) -> ()  [unwired: 2 in, 2 out]
        n32 = property on="校准模式" class="Enum (严格)"("DisabledEnum"=w63) -> ()  [unwired: 2 in, 2 out]
        n33 = Increment(x=w73) -> (x+1=w71:i32)
        n34 = global read "多参数全局变量.vi" "多参数编号"() -> (w76:string)
        n35 = Format Into String(format string="编号：%s\n参数：%s\n信息：%s%d%s" ("格式字符串"), w76, w74, "正在进行第" ("消息"), w71, "点校准，请放置好标液后按确认键继续。" ("消息")) -> (resulting string=w68:string)  [unwired: 2 in, 1 out]
        n36 = Two Button Dialog(message=w68) -> (T button?=w67:bool)  [unwired: 2 in]
        n37 = call "Add State to Queue.vi"("State(s) In (\"\")"="init: all\nCal: Over\nidle" ("State(s) In (\"\")")) -> ("States Out"=w66:string)  [unwired: 14 in]
        n38 = Select(t=w65, s=w67, f=w66) -> (s? t:f=w64:string)
      }
      frame "Cal: Calibration process" {
        # "进入此流程60秒后判断测量值最大值与最小值，如果小于2，则认为数据稳定，可以写入校准数据，如果超过180秒未通过校准，认为校准异常，停止校准"
        n39 = case shown="1" w80 {
          frame 0, Default {
          }
          frame 1 {
            n40 = local read "偏移值补偿"() -> (w102:dbl)
            n41 = Not Equal To 0?(x=w102) -> (x != 0?=w103:bool)
            n42 = case shown="真" w103 {
              frame False {
              }
              frame True {
                n43 = property on="偏移值补偿" class="DigNum (严格)"("Val(Sgnl)"=0.0 ("值(信号)")) -> ()  [unwired: 2 in, 2 out]
              }
            }
          }
        }
        n44 = local read "最大值"() -> (w100:sgl)
        n45 = local read "最小值"() -> (w99:sgl)
        n46 = Subtract(x=w100, y=w99) -> (x-y=w101:sgl)
        n47 = call "已用时间"("Reset"=w83) -> ("Elapsed Time (s)"=w79:dbl, "Time has Elapsed"=w97:bool)  [unwired: 11 in, 6 out]
        n48 = Greater Or Equal?(x=w79, y=120.0) -> (x >= y?=w92:bool)
        n49 = Less Or Equal?(x=w101, y=2.0) -> (x <= y?=w88:bool)
        n50 = And(x=w92, y=w88) -> (x .and. y?=w89:bool)
        n51 = Select(t="Cal: Calibration successful" ("State(s) In (\"\")"), s=w89, f="idle\nCal: Calibration process" ("State(s) In (\"\")")) -> (s? t:f=w87:string)
        n52 = Wait (ms)(milliseconds to wait=u32 100 ("等待时间（毫秒）")) -> ()  [unwired: 1 out]
        n53 = Select(t="Cal: Calibration failed" ("State(s) In (\"\")"), s=w97, f=w87) -> (s? t:f=w86:string)
        n54 = call "Add State to Queue.vi"("State(s) In Front (\"\")"=w86, "State(s) In (\"\")"=w96) -> ("States Out"=w95:string)  [unwired: 13 in]
        n55 = Format Into String(format string="正在进行第%d点校准，此过程可能需要几分钟，请耐性等待，已进行%d秒。" ("格式字符串"), w80, w79) -> (resulting string=→"提示":string)  [unwired: 2 in, 1 out]
      }
      frame "Cal: Calibration successful" {
        n56 = local read "测量读值"() -> (w108:dbl)
        n57 = local read "饱和度值"() -> (w109:dbl)
        n58 = case shown="\"两点校准\", 默认" w105 {
          tunnel: [w128 w137] -> w114
          tunnel: [w127 "Cal: Pass" ("State(s) In (\"\")")] -> w113
          tunnel: w106 -> [w126 _]
          frame "两点校准", Default {
            n59 = case shown="2, 默认" w126 {
              tunnel: [w129 w133] -> w128
              tunnel: ["Cal: Pass" ("State(s) In (\"\")") "Cal: Place standard solution\n Cal: Calibration process" ("State(s) In (\"\")")] -> w127
              frame 2, Default {
                n60 = global read "多参数全局变量.vi" "MB session in"() -> (w130:refnum<class "MB_Master.lvclass">)
                n61 = call "0032H_DO_第二点校正指令写入.vi"("数值"=u16 33, "MB session in"=w130) -> ("error out"=w129:errorcluster)  [unwired: 8 in, 1 out]
              }
              frame 1 {
                n62 = global read "多参数全局变量.vi" "MB session in"() -> (w134:refnum<class "MB_Master.lvclass">)
                n63 = call "002FH_DO_第一点校正指令写入.vi"("数值"=u16 17, "MB session in"=w134) -> ("error out"=w133:errorcluster)  [unwired: 8 in, 1 out]
              }
            }
          }
          frame "单点校准" {
            n64 = global read "多参数全局变量.vi" "MB session in"() -> (w139:refnum<class "MB_Master.lvclass">)
            n65 = call "0032H_DO_第二点校正指令写入.vi"("数值"=u16 33, "MB session in"=w139) -> ("error out"=w137:errorcluster)  [unwired: 8 in, 1 out]
          }
        }
        n66 = case shown="2" w106 {
          tunnel: w109 -> [_ w116 w118]
          tunnel: w108 -> [_ w115 w117]
          frame 0, Default {
          }
          frame 1 {
            "第一点信号值" <- w116
            "第一点校准值" <- w115
          }
          frame 2 {
            "第二点信号值" <- w118
            "第二点校准值" <- w117
          }
        }
        n67 = case shown="错误" w114 {
          tunnel: w113 -> [w120 _]
          tunnel: [w120 "Cal: Calibration failed" ("State(s) In (\"\")")] -> w110
          tunnel: w106 -> [w119 _]
          frame No Error {
            n68 = flat-sequence {
              tunnel: w119 -> [w121]
              frame #0 {
                n69 = Format Into String(format string="第%d点校准通过，按确认继续。" ("格式字符串"), w121) -> (resulting string=w123:string)  [unwired: 2 in, 1 out]
                n70 = One Button Dialog(message=w123) -> ()  [unwired: 1 in, 1 out]
              }
              frame #1 {
                n71 = Wait (ms)(milliseconds to wait=u32 2000 ("等待时间（毫秒）")) -> ()  [unwired: 1 out]
              }
            }
          }
          frame Error {
          }
        }
        n72 = call "Add State to Queue.vi"("State(s) In Front (\"\")"=w110, "State(s) In (\"\")"=w112) -> ("States Out"=w111:string)  [unwired: 13 in]
      }
      frame "Cal: Calibration failed" {
        n73 = global read "多参数全局变量.vi" "多参数编号"() -> (w145:string)
        n74 = call "Add State to Queue.vi"("State(s) In (\"\")"="init: all\nCal: Over\nidle" ("State(s) In (\"\")")) -> ("States Out"=w148:string)  [unwired: 14 in]
        n75 = Format Into String(format string="编号：%s\n参数：%s\n信息：%s" ("格式字符串"), w145, w142, "校准失败！" ("消息")) -> (resulting string=w144:string)  [unwired: 2 in, 1 out]
        n76 = One Button Dialog(message=w144) -> ()  [unwired: 1 in, 1 out]
        n77 = call "校准日志.vi"("table"="校准记录", "日志信息"=w144) -> ()  [unwired: 9 in, 1 out]
      }
      frame "Cal: Pass" {
        n78 = flat-sequence {
          tunnel: [w169] -> w157
          tunnel: w156 -> [w168]
          tunnel: [w167] -> w154
          tunnel: [w166] -> w153
          frame #0 {
            n79 = Wait (ms)(milliseconds to wait=u32 3000 ("等待时间（毫秒）")) -> ()  [unwired: 1 out]
          }
          frame #1 {
            n80 = global read "国弘过程全局变量.vi" "DO"() -> (w170:T2)
            n81 = Unbundle By Name(w170) -> ("电极状态标志"=w171:u16, "溶解氧电极零点"=w167:sgl, "溶解氧电极斜率"=w166:sgl)
            n82 = case shown="\"两点校准\", 默认" w168 {
              tunnel: [w177 w181] -> w169
              tunnel: w171 -> [_ _]
              frame "两点校准", Default {
                n83 = local read "第一点校准值"() -> (w175:dbl)
                n84 = local read "第一点信号值"() -> (w176:dbl)
                n85 = local read "第二点信号值"() -> (w172:dbl)
                n86 = local read "第二点校准值"() -> (w173:dbl)
                n87 = Format Into String(format string="校准结果：\n第一点校准值=%#.2f，第一点信号值=%#.2f mV，第一点标准值=0 %%；\n第二点校准值=%#.2f，第二点信号值=%#.2f mV，第二点标准值=100 %%。" ("提示"), w175, w176, w173, w172) -> (resulting string=w177:string)  [unwired: 2 in, 1 out]
              }
              frame "单点校准" {
                n88 = local read "第一点校准值"() -> (w180:dbl)
                n89 = local read "第一点信号值"() -> (w178:dbl)
                n90 = Format Into String(format string="校准结果：\n校准值=%#.2f，信号值=%#.2f，标准值=100 %%。" ("提示"), w180, w178) -> (resulting string=w181:string)  [unwired: 2 in, 1 out]
              }
            }
          }
        }
        n91 = call "Add State to Queue.vi"("State(s) In (\"\")"="init: all\nCal: Over\nidle" ("State(s) In (\"\")")) -> ("States Out"=w155:string)  [unwired: 14 in]
        n92 = global read "多参数全局变量.vi" "多参数编号"() -> (w161:string)
        n93 = Format Into String(format string="编号：%s\n参数：%s\n信息：%s\n电极零点=%#.2f%%，电极斜率=%#.2f%%" ("格式字符串"), w161, w160, w157, w154, w153) -> (resulting string=w158:string)  [unwired: 2 in, 1 out]
        n94 = One Button Dialog(message=w158) -> ()  [unwired: 1 in, 1 out]
        n95 = call "校准日志.vi"("table"="校准记录", "日志信息"=w158) -> ()  [unwired: 9 in, 1 out]
      }
      frame "Cal: Over" {
        n96 = global read "多参数全局变量.vi" "校准运行状态"() -> (w183:T4)
        n97 = Bundle By Name(cluster=w183, "DO"=FALSE) -> (w184:T4)
        n98 = global write "多参数全局变量.vi" "校准运行状态"(w184) -> ()
      }
      frame "idle", Default {
        n99 = event shown="[8] \"校准启动\": 值改变" {
          selector: _ -> [_ _ _ _ _ _ _ _ _ _]
          dyn-events: _ -> [_ _ _ _ _ _ _ _ _ _]
          timeout: 10 -> [_ _ _ _ _ _ _ _ _ _]
          tunnel: [_ _ _ _ w241 w247 w253 _ _ _] -> _
          tunnel: w195 -> [w210 w214 w217 w226 w240 w246 w252 w260 w271 _]
          tunnel: [w209 w213 w218 w227 w244 w250 w256 w259 w270 w273] -> w194
          tunnel: [w208 w211 w219 w228 w245 w251 w257 w258 w268 w274] -> w193
          tunnel: w192 -> [w208 w211 w219 w228 w245 w251 w257 w258 w268 w274]
          event Timeout {
            n100 = event-data() -> ()  [unwired: 1 in, 3 out]
            n101 = global read "国弘过程全局变量.vi" "DO"() -> (w196:T2)
            n102 = Unbundle By Name(w196) -> ("溶解氧电极零点"=→"电极零点":sgl, "溶解氧电极斜率"=→"电极斜率":sgl, "大气压补偿值"=→"气压补偿值":sgl, "盐度补偿值"=→"盐度补偿值":sgl, "溶解氧偏移修正值"=→"偏移值补偿":sgl, "溶解氧饱和度值"=→"饱和度值":sgl, "溶解氧测量值"=→"测量读值":sgl)  [unwired: 1 out]
            n103 = global read "多参数全局变量.vi" "DO通讯状态"() -> (w207:bool)
            n104 = property on="通讯状态" class="Str"("Blinking"=TRUE ("闪烁"), "Text.BG Color"=u32 16711680, "Visible"=w207) -> ()  [unwired: 2 in, 2 out]
            n105 = call "Add State to Queue.vi"("State(s) In (\"\")"=w210) -> ("States Out"=w209:string)  [unwired: 14 in]
            "通讯状态" <- "通讯异常" ("当前串口")
          }
          event "校准模式": Value Change {
            n106 = event-data() -> ()  [unwired: 1 in, 6 out]
            n107 = call "Add State to Queue.vi"("State(s) In (\"\")"=w214, "State(s) At Back (\"\")"="init: all\nidle" ("State(s) In (\"\")")) -> ("States Out"=w213:string)  [unwired: 13 in]
          }
          event "气压补偿值", "偏移值补偿": Mouse Down {
            n108 = event-data() -> ("CtlRef"=w216:refnum<vi>)  [unwired: 1 in, 7 out]
            n109 = property class="DigNum (严格)"(reference=w216) -> ("DisabledEnum"=w215:T3)  [unwired: 1 in, 2 out]
            n110 = case shown="\"Enabled\"" w215 {
              tunnel: w216 -> [w223 _]
              frame "Enabled" {
                n111 = property class="DigNum (严格)"(reference=w223) -> (reference out=w220:refnum<vi>, "Value"=w221:dbl)  [unwired: 1 in, 1 out]
                n112 = call "数字键盘.vi"("OldNumber"=w221) -> ("NewNumber"=w222:dbl)  [unwired: 1 in]
                n113 = property class="DigNum (严格)"(reference=w220, "Val(Sgnl)"=w222) -> ()  [unwired: 1 in, 2 out]
              }
              frame "Disabled", Default {
              }
            }
            n114 = call "Add State to Queue.vi"("State(s) In (\"\")"=w217) -> ("States Out"=w218:string)  [unwired: 14 in]
          }
          event "盐度补偿值": Mouse Down {
            n115 = event-data() -> ("CtlRef"=w225:refnum<vi>)  [unwired: 1 in, 7 out]
            n116 = property class="DigNum (严格)"(reference=w225) -> ("DisabledEnum"=w224:T3)  [unwired: 1 in, 2 out]
            n117 = case shown="\"Enabled\"" w224 {
              tunnel: w225 -> [w237 _]
              frame "Enabled" {
                n118 = global read "断电保存变量.vi" "Cond"() -> (w229:bool)
                n119 = case shown="真" w229 {
                  tunnel: [_ w238] -> w234
                  frame False {
                  }
                  frame True {
                    n120 = Two Button Dialog(message="是否使用系统测试值自动补偿" ("消息")) -> (T button?=w238:bool)  [unwired: 2 in]
                  }
                }
                n121 = global read "多参数全局变量.vi" "盐度显示"() -> (w233:cluster{"温度测量值":sgl, "测量值":sgl, "温度偏移修正值":sgl})
                n122 = Unbundle By Name(w233) -> ("测量值"=w232:sgl)
                n123 = property class="DigNum (严格)"(reference=w237) -> (reference out=w235:refnum<vi>, "Value"=w231:dbl)  [unwired: 1 in, 1 out]
                n124 = Select(t=w232, s=w234, f=w231) -> (s? t:f=w230:dbl)
                n125 = call "数字键盘.vi"("OldNumber"=w230) -> ("NewNumber"=w236:dbl)  [unwired: 1 in]
                n126 = property class="DigNum (严格)"(reference=w235, "Val(Sgnl)"=w236) -> ()  [unwired: 1 in, 2 out]
              }
              frame "Disabled", Default {
              }
            }
            n127 = call "Add State to Queue.vi"("State(s) In (\"\")"=w226) -> ("States Out"=w227:string)  [unwired: 14 in]
          }
          event "盐度补偿值": Value Change {
            n128 = event-data() -> ("NewVal"=w242:dbl)  [unwired: 1 in, 5 out]
            n129 = global read "多参数全局变量.vi" "MB session in"() -> (w243:refnum<class "MB_Master.lvclass">)
            n130 = call "0008H_DO_盐度补偿值写入.vi"("数值"=w242, "MB session in"=w243) -> ("error out"=w241:errorcluster)  [unwired: 8 in, 1 out]
            n131 = call "Add State to Queue.vi"("State(s) In (\"\")"=w240) -> ("States Out"=w244:string)  [unwired: 14 in]
          }
          event "气压补偿值": Value Change {
            n132 = event-data() -> ("NewVal"=w248:dbl)  [unwired: 1 in, 5 out]
            n133 = global read "多参数全局变量.vi" "MB session in"() -> (w249:refnum<class "MB_Master.lvclass">)
            n134 = call "000AH_DO_大气压补偿值写入.vi"("数值"=w248, "MB session in"=w249) -> ("error out"=w247:errorcluster)  [unwired: 8 in, 1 out]
            n135 = call "Add State to Queue.vi"("State(s) In (\"\")"=w246) -> ("States Out"=w250:string)  [unwired: 14 in]
          }
          event "偏移值补偿": Value Change {
            n136 = event-data() -> ("NewVal"=w254:dbl)  [unwired: 1 in, 5 out]
            n137 = global read "多参数全局变量.vi" "MB session in"() -> (w255:refnum<class "MB_Master.lvclass">)
            n138 = call "000CH_DO_DO偏移修正值写入.vi"("数值"=w254, "MB session in"=w255) -> ("error out"=w253:errorcluster)  [unwired: 8 in, 1 out]
            n139 = call "Add State to Queue.vi"("State(s) In (\"\")"=w252) -> ("States Out"=w256:string)  [unwired: 14 in]
          }
          event "刷新按钮": Value Change {
            n140 = event-data() -> ()  [unwired: 1 in, 6 out]
            n141 = call "Add State to Queue.vi"("State(s) In (\"\")"=w260) -> ("States Out"=w259:string)  [unwired: 14 in]
            n142 = Two Button Dialog(message="请再次确实是否恢复出厂设置！" ("消息")) -> (T button?=w262:bool)  [unwired: 2 in]
            n143 = case shown="真" w262 {
              frame False {
              }
              frame True {
                w263 = u16 33 items=["Factory Reset"=33] ("数值")
                n144 = global read "多参数全局变量.vi" "MB session in"() -> (w264:refnum<class "MB_Master.lvclass">)
                n145 = call "0026H_DO_命令寄存器写入.vi"("数值"=w263, "MB session in"=w264) -> ()  [unwired: 8 in, 2 out]
              }
            }
          }
          event "校准启动": Value Change {
            n146 = event-data() -> ()  [unwired: 1 in, 6 out]
            n147 = global read "多参数全局变量.vi" "校准运行状态"() -> (w266:T4)
            n148 = call "Add State to Queue.vi"("State(s) In (\"\")"=w271, "State(s) At Back (\"\")"="init: all\nCal: Place standard solution\n Cal: Calibration process\nidle" ("State(s) In (\"\")")) -> ("States Out"=w270:string)  [unwired: 13 in]
            n149 = Bundle By Name(cluster=w266, "DO"=TRUE) -> (w267:T4)
            n150 = global write "多参数全局变量.vi" "校准运行状态"(w267) -> ()
          }
          event "校准停止": Value Change {
            n151 = event-data() -> ()  [unwired: 1 in, 6 out]
            n152 = call "Add State to Queue.vi"("State(s) In (\"\")"="init: all\nCal: Over\nidle" ("State(s) In (\"\")")) -> ("States Out"=w273:string)  [unwired: 14 in]
          }
        }
      }
    }
  }
  n153 = while {
    stop <- FALSE stop-if-true
    n154 = global read "多参数全局变量.vi" "权限"() -> (w278:enum16{"一级权限", "二级权限", "三级权限"})
    n155 = Wait (ms)(milliseconds to wait=u32 1000 ("等待时间（毫秒）")) -> ()  [unwired: 1 out]
    n156 = Not Equal?(x=w278, y=enum16{"一级权限", "二级权限", "三级权限"}."一级权限") -> (x != y?=w276:bool)
    n157 = property on="偏移值补偿" class="DigNum (严格)"("Visible"=w276) -> ()  [unwired: 2 in, 2 out]
  }
